vi "Handle.vi"(8 "error in (no error)":errorcluster, 11 "uErr in":refnum<class "uErr.lvclass">) -> (0 "error out":errorcluster, 3 "uErr out":refnum<class "uErr.lvclass">)   [LabVIEW 2023, in "uLib.lvlib" / "uErr.lvclass"]
doc: "Dynamic dispatch method to enable children to define the error handling behavior. By default, this parent method does nothing."
uses:
  uErr.lvclass
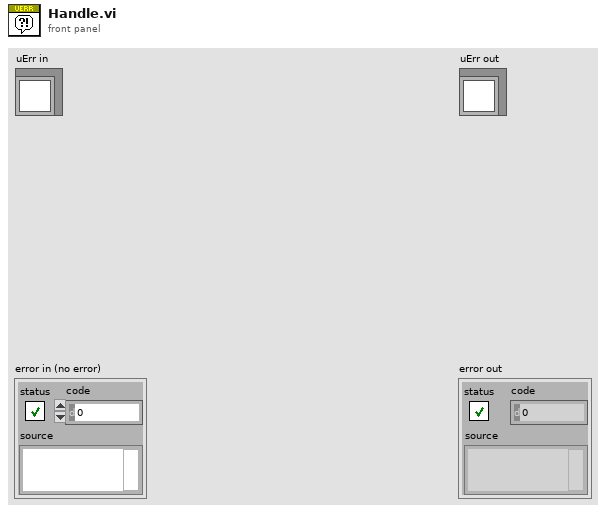
[diagram p1: front panel]
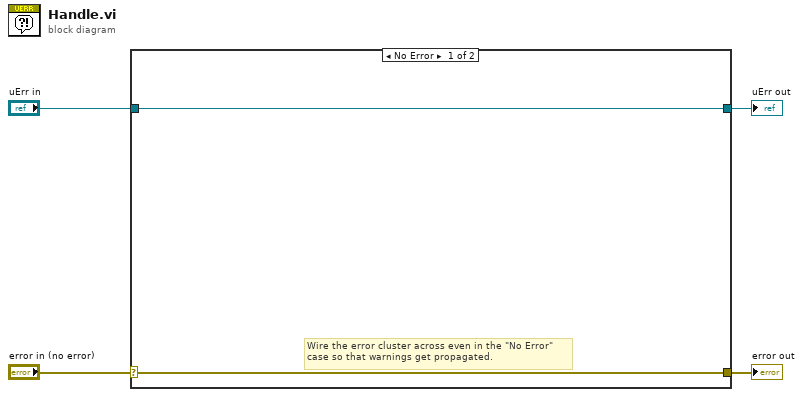
[diagram p0: block diagram]
diagram:
  n1 = case shown="No Error" "error in (no error)" {
    selector: "error in (no error)" -> [w5 w8]
    tunnel: [w5 w8] -> w3
    tunnel: [w6 w7] -> w1
    tunnel: "uErr in" -> [w6 w7]
    frame No Error {
      # "Wire the error cluster across even in the \"No Error\"\ncase so that warnings get propagated."
    }
    frame Error {
    }
  }
  "error out" <- w3
  "uErr out" <- w1
